vi "运维调试_CODCr.vi"() -> ()   [LabVIEW 2016, in "CODCr库.lvlib"]
uses:
  <vilib>/Utility/miscctls.llb/LVPointTypeDef.ctl
  <vilib>/Plasmionique/MB Master/MB_Master_Serial/MB_Master_Serial.lvclass
  D:/Program Files (x86)/National Instruments/LabVIEW 2016/vi.lib/Plasmionique/MB Master/MB_Master/MB_Master.lvclass
  <vilib>/Plasmionique/MB Master/MB Master.lvlib
  <vilib>/ptbypt/NI_PtbyPt.lvlib
  <vilib>/Utility/config.llb/NI_LVConfig.lvlib
panel:
  in  "加标回收测试":bool
  in  "平行样测试":bool
  in  "定时启动":bool
  out "COM口":string
  in  "空白测试":bool
  in  "隐藏按钮":bool
  in  "写入消解温度时长":bool
  in  "保存KB值":bool
  out "source":string
  in  "标样核查":bool
  out "启动时间":timestamp format="%<%Y/%m/%d %H:%M:%S>T"
  out "主循环次数":i32
  out "status":bool
  out "启动测量模式":T1(ring)
  out "曲线斜率B":sgl format="%#_10g"
  out "曲线斜率K":sgl format="%#_10g"
  out "量程上限":sgl
  out "量程下限":sgl
  out "消解时长":u16
  out "消解温度":u16
  out "测量精度":u16
  out "测量结果":sgl
  out "标样参考值":sgl
  out "量程":u16
  out "工作状态":T1(ring)
  out "仪器时间":timestamp format="%<%X\n%x>T"
  out "关键参数区":T2
  out "状态告警区":T3
  out "测量数据区":T4 {"单位" items=["ug/L", "mg/L", "ppm", "mg/m3", "cm", "ppb", "ug/m3", "%", "nmol/mol", "umol/mol", "MPN/L", "MPN/100ml", "ng/m3", "NTU", "无量纲", "ms/cm", "us/cm", "℃", "mV", "万个/L"]}
  out "系统时间":timestamp format="%<%Y/%m/%d %H:%M:%S>T"
  in  "VISA Resource":refnum<visa-resource-name>="COM9"
  out "Registers":u16[](array[numeric])
  in  "枚举":enum16{"读取", "写入", "读取参数"}(ring)
  in  "停止":bool
  in  "校时":bool
  in  "标样校准":bool
  in  "空白校准":bool
  in  "零点核查":bool
  in  "跨度核查":bool
  in  "水样测试":bool
  in  "返回":bool
  in  "设置":bool
  # "mg/L"
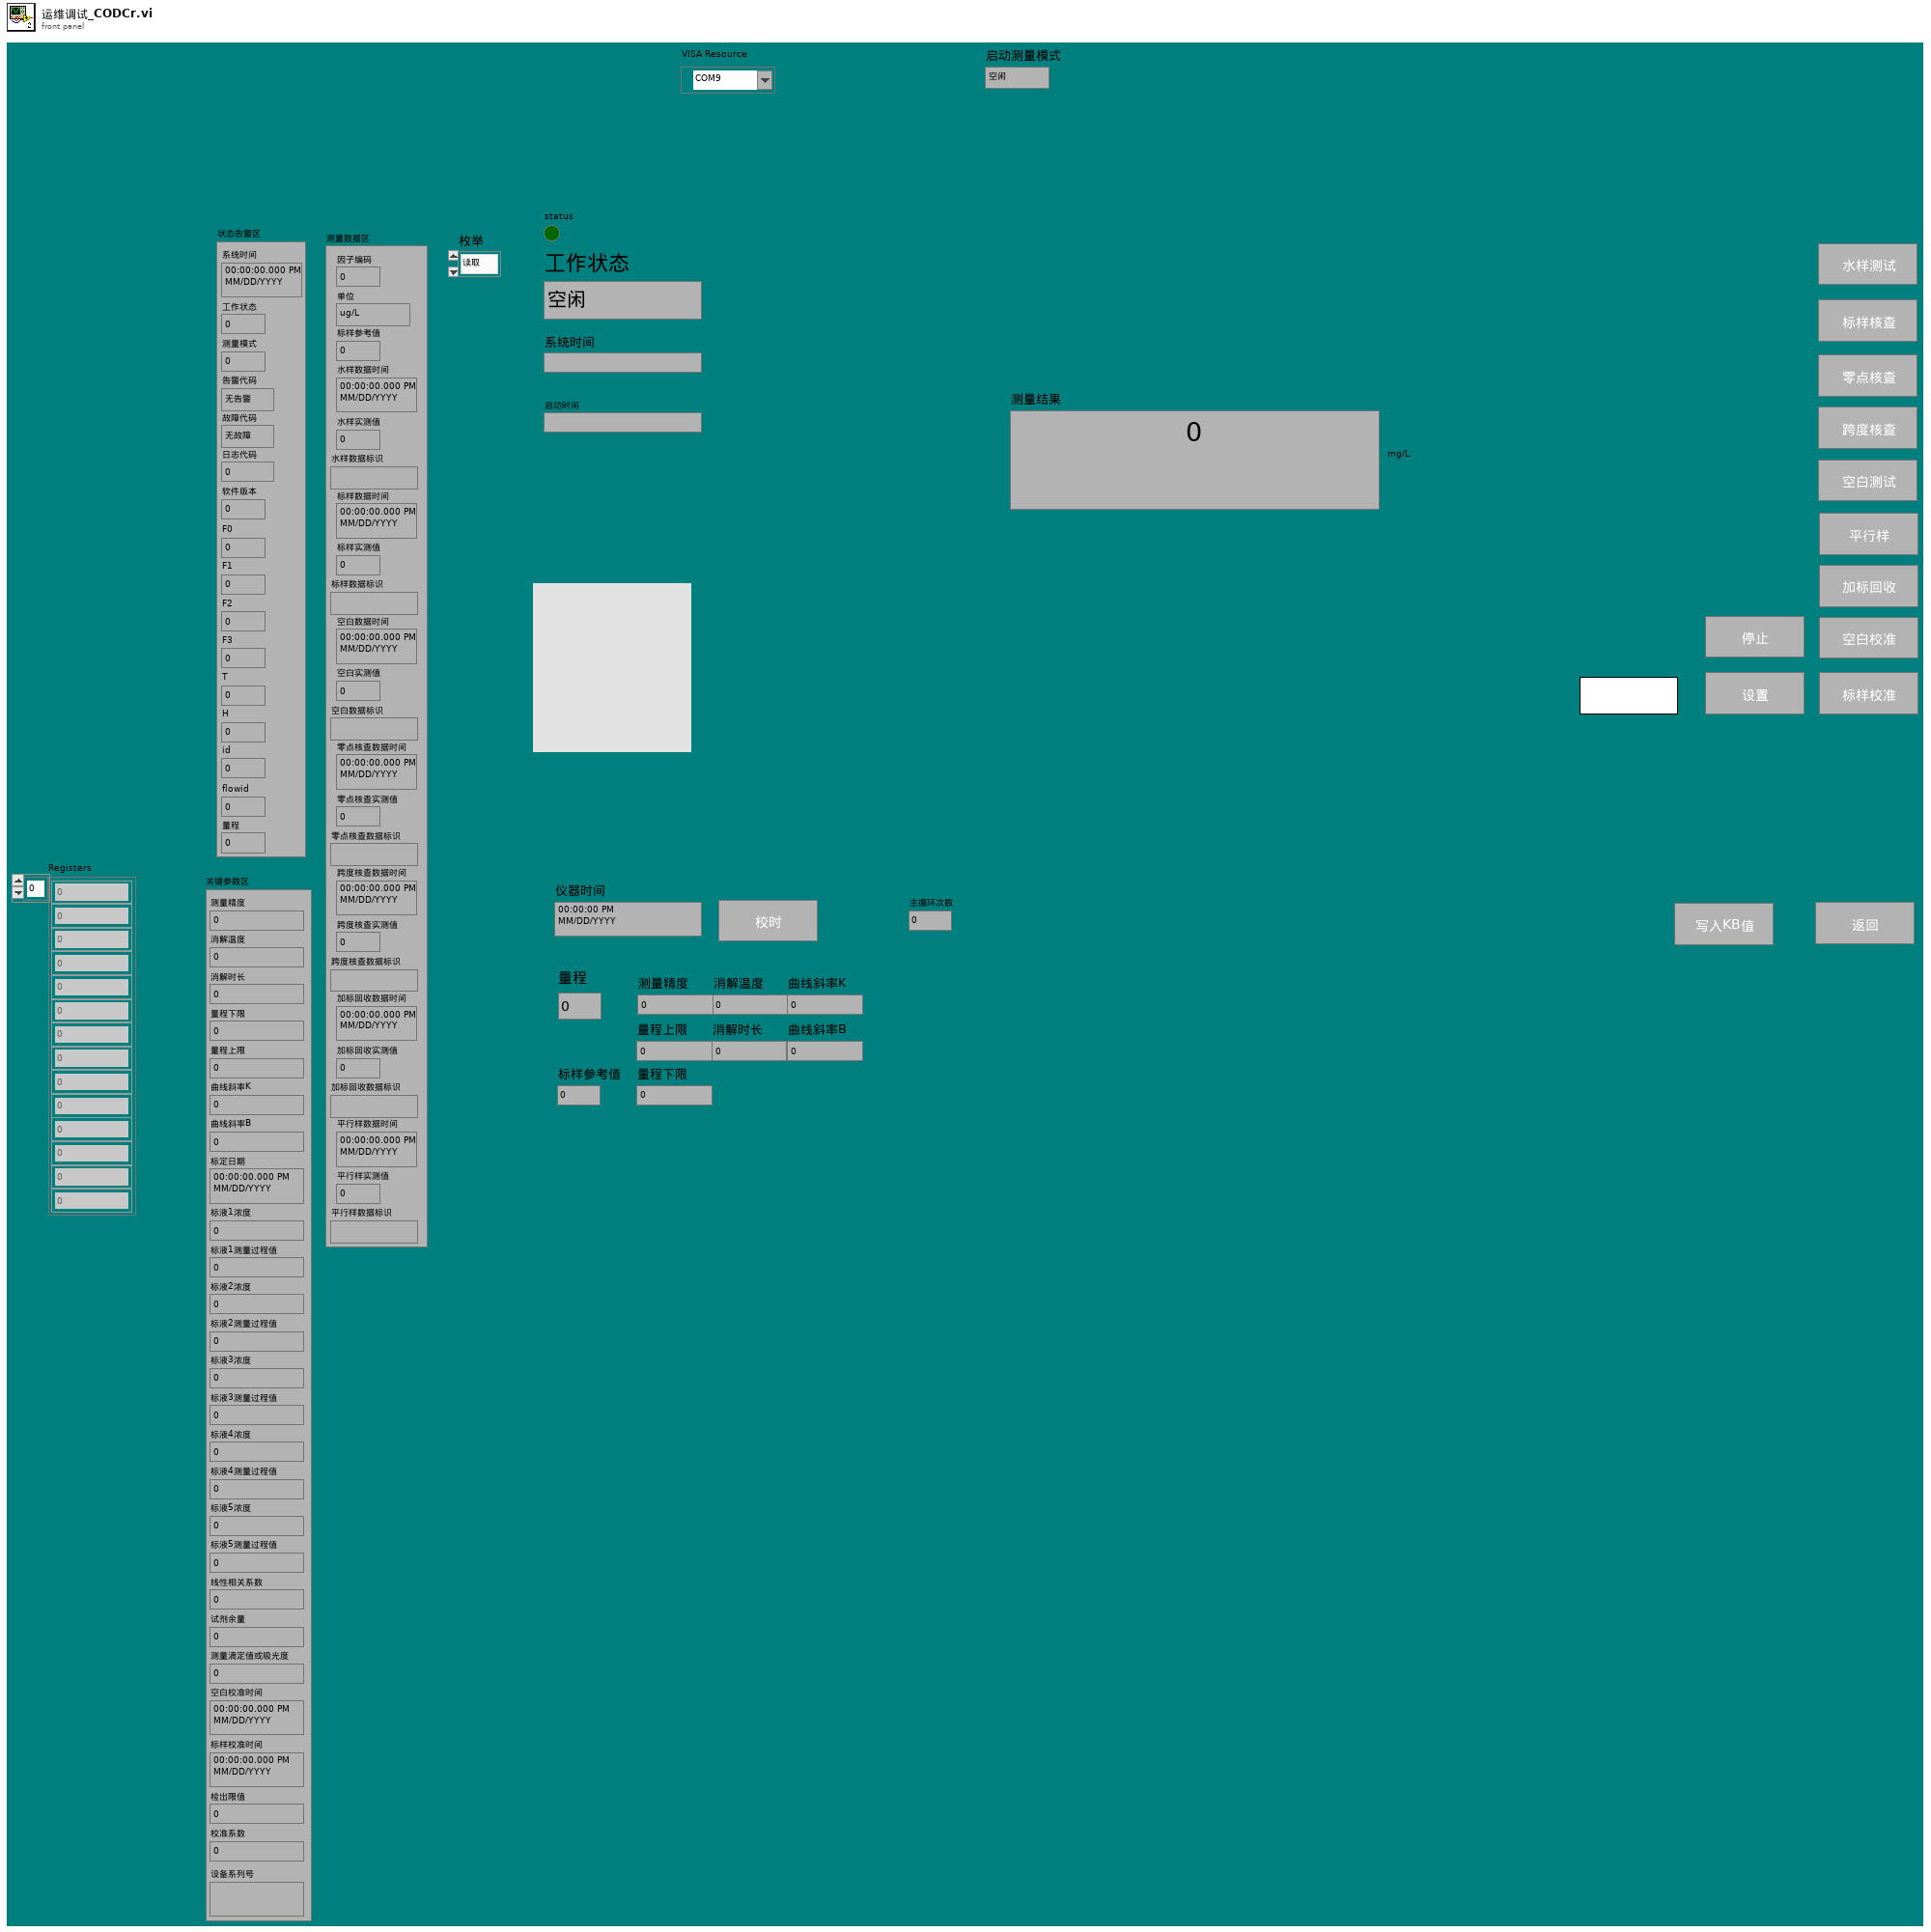
[diagram p1: front panel]
types:
  T1 = enum16{"空闲", "水样测试", "标样核查", "零点核查", "跨度核查", "空白测试", "平行样测试", "加标回收", "空白校准", "标样校准", "初始化（清洗）"}
  T2 = cluster{"测量精度":u16, "消解温度":u16, "消解时长":u16, "量程下限":sgl, "量程上限":sgl, "曲线斜率K":sgl, "曲线斜率B":sgl, "标定日期":timestamp, "标液1浓度":sgl, "标液1测量过程值":sgl, "标液2浓度":sgl, "标液2测量过程值":sgl, "标液3浓度":sgl, "标液3测量过程值":sgl, "标液4浓度":sgl, "标液4测量过程值":sgl, "标液5浓度":sgl, "标液5测量过程值":sgl, "线性相关系数":sgl, "试剂余量":u32, "测量滴定值或吸光度":sgl, "空白校准时间":timestamp, "标样校准时间":timestamp, "检出限值":sgl, "校准系数":sgl, "设备系列号":string}
  T3 = cluster{"系统时间":timestamp, "工作状态":u16, "测量模式":u16, "告警代码":enum16{"无告警", "缺试剂告警", "缺水样告警", "缺蒸馏水告警", "缺标液告警", "仪表漏液告警", "标定异常告警", "超量程告警", "加热异常", "低试剂预警", "超上限告警", "超下限告警", "仪表内部其他异常", "滴定异常告警", "电极异常告警", "量程切换告警", "参数设置告警", "PH电极电位异常", "电导率电极异常", "浊度光度异常", "溶解氧电极异常", "溶解氧光强异常", "温度异常告警", "PH异常告警", "溶解氧异常告警", "电导率异常告警", "浊度异常告警", "叶绿素异常告警", "藻密度异常告警", "蓝绿藻异常告警", "ORP异常告警", "氨氮异常告警", "清洁刷异常告警", "SD卡异常告警", "蓝牙异常告警", "Wifi异常告警", "流程异常告警"}, "故障代码":enum16{"无故障", "电机故障", "温度故障", "通讯故障", "滴定故障"}, "日志代码":u16, "软件版本":u16, "F0":sgl, "F1":sgl, "F2":sgl, "F3":sgl, "T":sgl, "H":sgl, "id":u16, "flowid":u16, "量程":u16}
  T4 = cluster{"因子编码":u32, "单位":u16, "标样参考值":sgl, "水样数据时间":timestamp, "水样实测值":sgl, "水样数据标识":string, "标样数据时间":timestamp, "标样实测值":sgl, "标样数据标识":string, "空白数据时间":timestamp, "空白实测值":sgl, "空白数据标识":string, "零点核查数据时间":timestamp, "零点核查实测值":sgl, "零点核查数据标识":string, "跨度核查数据时间":timestamp, "跨度核查实测值":sgl, "跨度核查数据标识":string, "加标回收数据时间":timestamp, "加标回收实测值":sgl, "加标回收数据标识":string, "平行样数据时间":timestamp, "平行样实测值":sgl, "平行样数据标识":string}
  T5 = cluster{"baud rate (bps)":u32, "stop bits":u16, "parity":u16, "flow control":u16, "timeout":u32, "retries":i32}
  T6 = cluster{"starting address":u16, "number of holding registers":u16}
  T7 = cluster{"测量模式":enum16{"水样测量", "标样核查", "零点核查", "跨度核查", "空白测试", "加标回收", "平行样", "校零", "校标"}}
  T8 = cluster{"仪器测试类型":enum16{"水样测试", "标样核查", "空白测试", "跨度核查"}, "周期设置类型":enum16{"定点启动", "间隔启动"}, "定时功能启用":bool, "定时间隔":dbl, "24H周期设置":bool[]}
  T9 = typedef "LVDateTimeRec.ctl" = cluster{"秒数的小数部分":dbl, "秒":i32, "分":i32, "时":i32, "日":i32, "月":i32, "年":i32, "天数（周）":i32, "天数（年）":i32, "DST":i32}
  T10 = typedef "LVPointTypeDef.ctl" = cluster{"Horizontal":i16, "Vertical":i16}
  T11 = typedef "NI_LVConfig.lvlib/Config Data RefNum.ctl" = refnum<k1>
  T12 = cluster{"运行模式":enum16{"维护模式", "常规模式", "应急模式", "质控模式"}}
  T13 = cluster{"时间标识":timestamp, "监测值":sgl, "单位":u16, "数据标识":string, "因子编码":u32, "标样参考值":sgl, "F0":sgl, "F1":sgl, "F2":sgl, "F3":sgl, "温度":sgl, "湿度":sgl, "量程标识":string}
  T14 = cluster{"系统时间":timestamp, "工作状态":enum16{"空闲", "水样测试", "标样核查", "零点核查", "跨度核查", "空白测试", "平行样测试", "加标回收", "空白校准", "标样校准", "初始化（清洗）"}, "测量模式":enum16{"待机", "连续模式", "周期模式", "定点模式", "受控模式", "手动模式"}, "告警代码":enum16{"无告警", "缺试剂告警", "缺水样告警", "缺蒸馏水告警", "缺标液告警", "仪表漏液告警", "标定异常告警", "超量程告警", "加热异常", "低试剂预警", "超上限告警", "超下限告警", "仪表内部其他异常", "滴定异常告警", "电极异常告警", "量程切换告警", "参数设置告警", "PH电极电位异常", "电导率电极异常", "浊度光度异常", "溶解氧电极异常", "溶解氧光强异常", "温度异常告警", "PH异常告警", "溶解氧异常告警", "电导率异常告警", "浊度异常告警", "叶绿素异常告警", "藻密度异常告警", "蓝绿藻异常告警", "ORP异常告警", "氨氮异常告警", "清洁刷异常告警", "SD卡异常告警", "蓝牙异常告警", "Wifi异常告警", "流程异常告警"}, "故障代码":enum16{"无故障", "电机故障", "温度故障", "通讯故障", "滴定故障"}, "日志代码":u16, "软件版本":u16, "F0":sgl, "F1":sgl, "F2":sgl, "F3":sgl, "T":sgl, "H":sgl, "id":u16, "flowid":u16, "量程":u16}
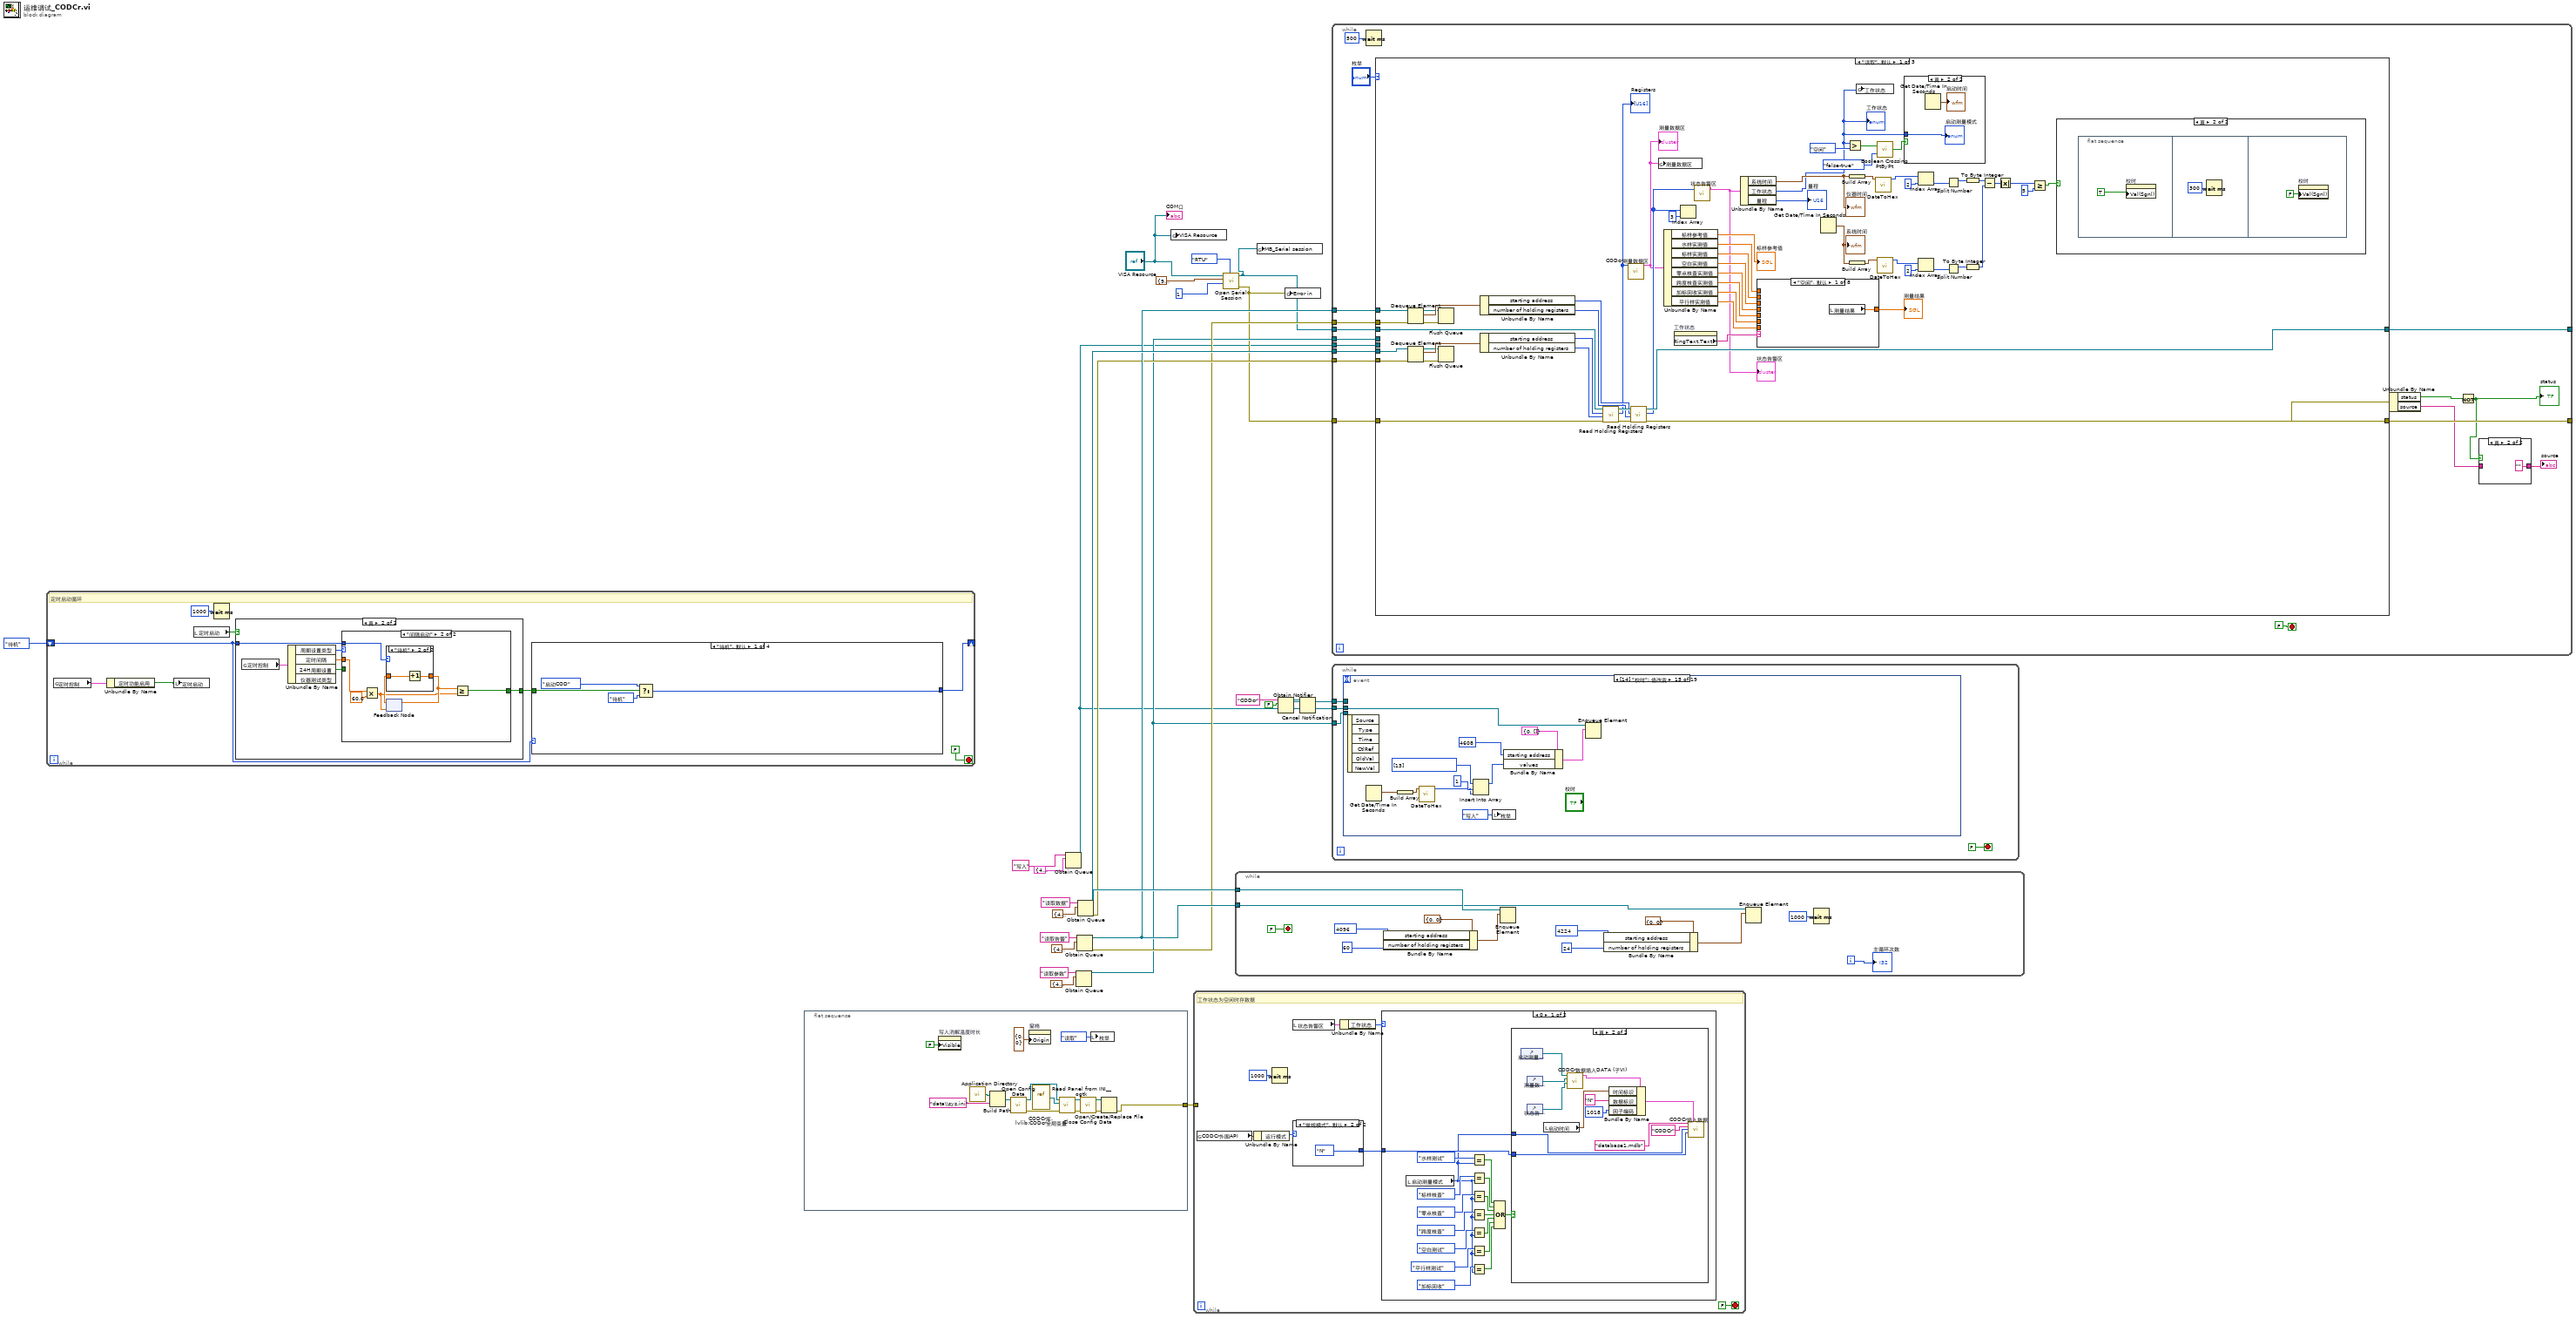
[diagram p0: block diagram]
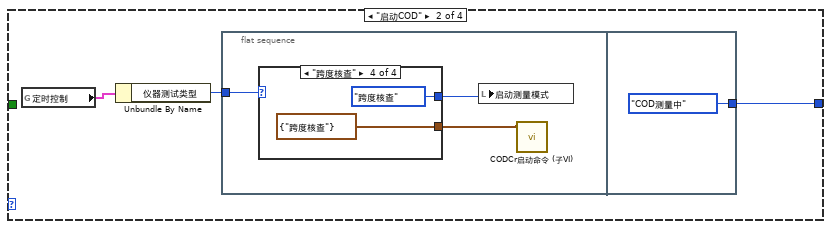
[diagram p2: hidden frame]
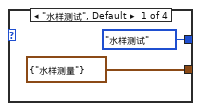
[diagram p3: hidden frame]
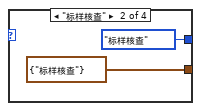
[diagram p4: hidden frame]
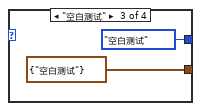
[diagram p5: hidden frame]
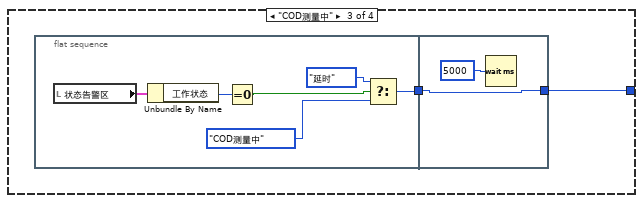
[diagram p6: hidden frame]
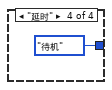
[diagram p7: hidden frame]
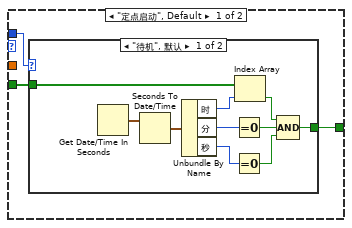
[diagram p9: hidden frame]
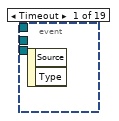
[diagram p12: hidden frame]
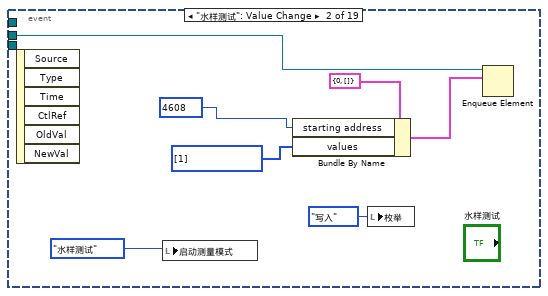
[diagram p13: hidden frame]
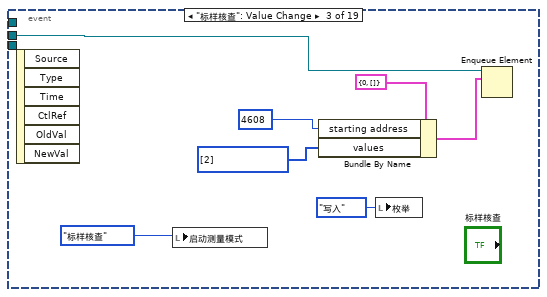
[diagram p14: hidden frame]
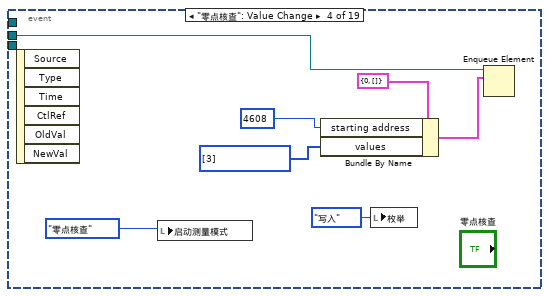
[diagram p15: hidden frame]
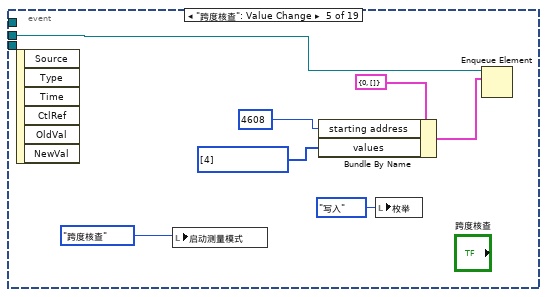
[diagram p16: hidden frame]
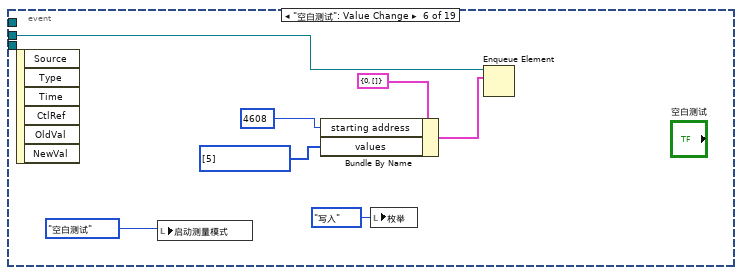
[diagram p17: hidden frame]
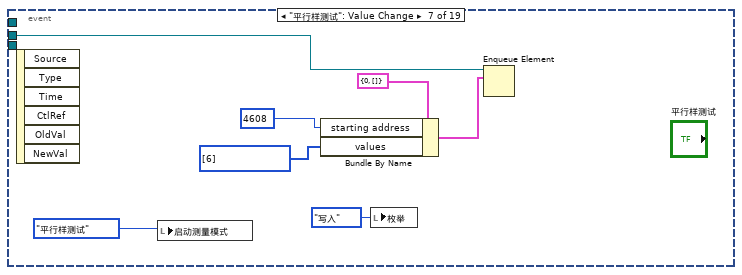
[diagram p18: hidden frame]
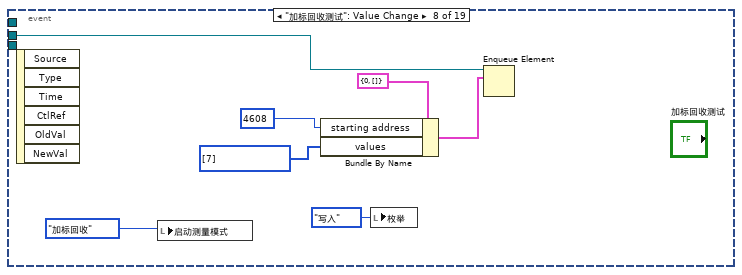
[diagram p19: hidden frame]
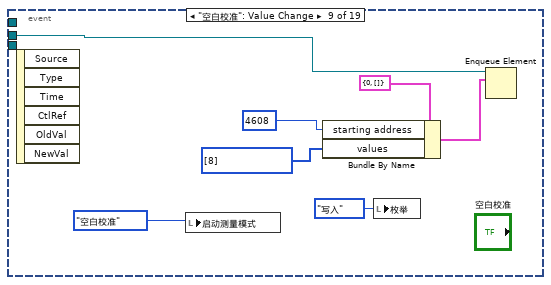
[diagram p20: hidden frame]
diagram:
  n1 = while {
    shift-right: [w32] -> _
    shift-left: enum16{"待机", "启动COD", "COD测量中", "延时"}."待机" -> [w31]
    stop <- FALSE stop-if-true
    # "定时启动循环"
    n2 = global read "CODcr全局变量.vi" "定时控制"() -> (w28:T8)
    n3 = Unbundle By Name(w28) -> ("定时功能启用"=w27:bool)
    n4 = local write "定时启动"(w27) -> ()
    n5 = local read "定时启动"() -> (w29:bool)
    n6 = Wait (ms)(milliseconds to wait=u32 1000 ("等待时间（毫秒）")) -> ()  [unwired: 1 out]
    n7 = case shown="真" w29 {
      tunnel: w31 -> [_ w67]
      tunnel: [_ w66] -> w30
      frame False {
      }
      frame True {
        n8 = global read "CODcr全局变量.vi" "定时控制"() -> (w65:T8)
        n9 = Unbundle By Name(w65) -> ("周期设置类型"=w68:enum16{"定点启动", "间隔启动"}, "定时间隔"=w69:dbl, "24H周期设置"=w70:bool[])  [unwired: 1 out]
        n10 = case shown="\"间隔启动\"" w68 {
          tunnel: w69 -> [_ w87]
          tunnel: w70 -> [w73 _]
          tunnel: w67 -> [w71 w90]
          tunnel: [w72 w85] -> w66
          frame "定点启动", Default {
            n11 = case shown="\"待机\", 默认" w71 {
              tunnel: w73 -> [w81 _]
              tunnel: [w74 _] -> w72
              frame "待机", Default {
                n12 = Get Date/Time In Seconds() -> (seconds since 1Jan1904=w83:timestamp)
                n13 = Seconds To Date/Time(time stamp (now)=w83) -> (date time rec=w82:T9)  [unwired: 1 in]
                n14 = Unbundle By Name(w82) -> ("时"=w80:i32, "分"=w78:i32, "秒"=w79:i32)
                n15 = Equal To 0?(x=w78) -> (x = 0?=w76:bool)
                n16 = Equal To 0?(x=w79) -> (x = 0?=w75:bool)
                n17 = Index Array(array=w81, index=w80) -> (element=w77:bool)
                n18 = Compound Arithmetic op=AND ("复合运算")(w77, w76, w75) -> (w74:bool)
              }
              frame "启动COD" {
              }
            }
          }
          frame "间隔启动" {
            n19 = Multiply(x=w87, y=60.0) -> (x*y=w84:dbl)
            n20 = feedback #1(w84) -> (w89:dbl)
            n21 = case shown="\"待机\"" w90 {
              tunnel: w89 -> [_ w92]
              tunnel: [_ w91] -> w88
              frame Default {
              }
              frame "待机" {
                n22 = Increment(x=w92) -> (x+1=w91:dbl)
              }
            }
            n23 = feedback-in #1(w88) -> ()
            n24 = Greater Or Equal?(x=w88, y=w84) -> (x >= y?=w85:bool)
          }
        }
      }
    }
    n25 = case shown="\"待机\", 默认" w31 {
      tunnel: [w35 w41 w55 enum16{"待机", "启动COD", "COD测量中", "延时"}."待机"] -> w32
      tunnel: w30 -> [w38 _ _ _]
      frame "待机", Default {
        n26 = Select(t=enum16{"待机", "启动COD", "COD测量中", "延时"}."启动COD", s=w38, f=enum16{"待机", "启动COD", "COD测量中", "延时"}."待机") -> (s? t:f=w35:enum16{"待机", "启动COD", "COD测量中", "延时"})
      }
      frame "启动COD" {
        n27 = global read "CODcr全局变量.vi" "定时控制"() -> (w39:T8)
        n28 = Unbundle By Name(w39) -> ("仪器测试类型"=w40:enum16{"水样测试", "标样核查", "空白测试", "跨度核查"})
        n29 = flat-sequence {
          tunnel: w40 -> [w44]
          tunnel: [enum16{"待机", "启动COD", "COD测量中", "延时"}."COD测量中"] -> w41
          frame #0 {
            n30 = case shown="\"跨度核查\"" w44 {
              tunnel: [T7 {"测量模式"=enum."水样测量"} ("启动测量模式") T7 {"测量模式"=enum."标样核查"} ("启动测量模式") T7 {"测量模式"=enum."空白测试"} ("启动测量模式") T7 {"测量模式"=enum."跨度核查"} ("启动测量模式")] -> w43
              tunnel: [T1."水样测试" ("启动测量模式") T1."标样核查" ("启动测量模式") T1."空白测试" ("启动测量模式") T1."跨度核查" ("启动测量模式")] -> w42
              frame "水样测试", Default {
              }
              frame "标样核查" {
              }
              frame "空白测试" {
              }
              frame "跨度核查" {
              }
            }
            n31 = local write "启动测量模式"(w42) -> ()
            n32 = call "CODCr启动命令 (子VI).vi"("启动测量模式"=w43) -> ()  [unwired: 11 in]
          }
          frame #1 {
          }
        }
      }
      frame "COD测量中" {
        n33 = flat-sequence {
          tunnel: [w59] -> w54
          tunnel: [w63] -> w55
          tunnel: w54 -> [w63]
          frame #0 {
            n34 = local read "状态告警区"() -> (w58:T3)
            n35 = Unbundle By Name(w58) -> ("工作状态"=w57:u16)
            n36 = Equal To 0?(x=w57) -> (x = 0?=w56:bool)
            n37 = Select(t=enum16{"待机", "启动COD", "COD测量中", "延时"}."延时", s=w56, f=enum16{"待机", "启动COD", "COD测量中", "延时"}."COD测量中") -> (s? t:f=w59:enum16{"待机", "启动COD", "COD测量中", "延时"})
          }
          frame #1 {
            n38 = Wait (ms)(milliseconds to wait=u32 5000 ("等待时间（毫秒）")) -> ()  [unwired: 1 out]
          }
        }
      }
      frame "延时" {
      }
    }
  }
  n39 = flat-sequence {
    tunnel: [w93] -> w1
    frame #0 {
      n40 = property on="写入消解温度时长" class="Bool"("Visible"=FALSE ("可见")) -> ()  [unwired: 2 in, 2 out]
      n41 = call <vilib>:"Application Directory.vi"() -> ("Application Directory"=w103:path)
      n42 = Build Path(base path=w103, name or relative path="data\\sys.ini" ("名称或相对路径")) -> (appended path=w101:path)
      n43 = call <vilib>:"Open Config Data.vi"("configuration file path"=w101) -> ("error out"=w97:errorcluster, "refnum"=w100:T11)  [unwired: 8 in, 1 out]
      n44 = property on="窗格" class="Pane"("Origin"=T10 {"Horizontal"=0, "Vertical"=0} ("原点")) -> ()  [unwired: 2 in, 2 out]
      n45 = vi-ref "CODCr库.lvlib:CODcr全局变量.vi"() -> (w99:refnum<vi>)
      n46 = call <userlib>:"Read Panel from INI__ogtk.vi"("error in (no error)"=w97, "VI ref"=w99, "refnum"=w100) -> ("error out"=w96:errorcluster, "refnum out"=w98:T11)  [unwired: 7 in]
      n47 = call <vilib>:"Close Config Data.vi"("error in (no error)"=w96, "refnum"=w98) -> ("error out"=w95:errorcluster, "file path"=w94:path)  [unwired: 8 in]
      n48 = local write "枚举"(enum16{"读取", "写入", "读取参数"}."读取" ("枚举")) -> ()
      n49 = Open/Create/Replace File(file path (use dialog)=w94, error in=w95) -> (error out=w93:errorcluster)  [unwired: 4 in, 2 out]
    }
  }
  n50 = Obtain Queue(name (unnamed)="写入" ("名称（未命名）"), element data type=cluster{"starting address":u16, "values":u16[]} {"starting address"=4096, "values"=[]}) -> (queue out=w3:refnum<queue>)  [unwired: 3 in, 2 out]
  n51 = Obtain Queue(name (unnamed)="读取参数" ("名称（未命名）"), element data type=T6 {"starting address"=4096, "number of holding registers"=100}) -> (queue out=w7:refnum<queue>)  [unwired: 3 in, 2 out]
  n52 = Obtain Queue(name (unnamed)="读取告警" ("名称（未命名）"), element data type=T6 {"starting address"=4096, "number of holding registers"=100}) -> (queue out=w16:refnum<queue>, error out=w12:errorcluster)  [unwired: 3 in, 1 out]
  n53 = Obtain Queue(name (unnamed)="读取数据" ("名称（未命名）"), element data type=T6 {"starting address"=4096, "number of holding registers"=100}) -> (queue out=w19:refnum<queue>, error out=w13:errorcluster)  [unwired: 3 in, 1 out]
  n54 = global write "CODcr全局变量.vi" "VISA Resource"("VISA Resource") -> ()
  n55 = while "While循环" {
    tunnel: w1 -> [_]
    stop <- FALSE stop-if-true
    # "工作状态为空闲时存数据"
    n56 = global read "CODCr外部API.vi" "CODCr外围API"() -> (w108:T12)
    n57 = Unbundle By Name(w108) -> ("运行模式"=w107:enum16{"维护模式", "常规模式", "应急模式", "质控模式"})
    n58 = Wait (ms)(milliseconds to wait=u32 1000 ("等待时间（毫秒）")) -> ()  [unwired: 1 out]
    n59 = local read "状态告警区"() -> (w111:T3)
    n60 = case shown="\"常规模式\", 默认" w107 {
      tunnel: [enum16{"N", "M"}."M" ("数据类型") enum16{"N", "M"}."N" ("数据类型")] -> w109
      frame "维护模式" {
      }
      frame "常规模式", Default {
      }
    }
    n61 = Unbundle By Name(w111) -> ("工作状态"=w110:u16)
    n62 = case shown="0" w110 {
      tunnel: w109 -> [w132 _]
      frame 0 {
        n63 = local read "启动测量模式"() -> (w124:T1)
        n64 = Equal?(x=T1."水样测试" ("启动测量模式"), y=w124) -> (x = y?=w123:bool)
        n65 = Equal?(x=T1."标样核查" ("启动测量模式"), y=w124) -> (x = y?=w122:bool)
        n66 = Equal?(x=T1."零点核查" ("启动测量模式"), y=w124) -> (x = y?=w121:bool)
        n67 = Equal?(x=T1."跨度核查" ("启动测量模式"), y=w124) -> (x = y?=w120:bool)
        n68 = Equal?(x=T1."空白测试" ("启动测量模式"), y=w124) -> (x = y?=w119:bool)
        n69 = Equal?(x=T1."平行样测试" ("启动测量模式"), y=w124) -> (x = y?=w118:bool)
        n70 = Equal?(x=T1."加标回收" ("启动测量模式"), y=w124) -> (x = y?=w117:bool)
        n71 = Compound Arithmetic op=OR(w123, w122, w121, w120, w119, w118, w117) -> (w116:bool)
        n72 = case shown="真" w116 {
          tunnel: w124 -> [_ w134]
          tunnel: w132 -> [_ w133]
          frame False {
          }
          frame True {
            n73 = control-ref of="启动测量模式"() -> (w141:refnum<vi>)
            n74 = control-ref of="测量数据区"() -> (w140:refnum<vi>)
            n75 = control-ref of="状态告警区"() -> (w139:refnum<vi>)
            n76 = local read "启动时间"() -> (w144:timestamp)
            n77 = call "CODCr数据插入DATA (子VI).vi"("reference 2"=w139, "reference"=w140, "Enum输入"=w141) -> ("data"=w138:T13)  [unwired: 8 in]
            n78 = Bundle By Name(cluster=w138, "时间标识"=w144, "数据标识"="N", "因子编码"=u32 1018) -> (w137:T13)
            n79 = call "CODCr插入数据.vi"("database"="database1.mdb", "data"=w137, "table"="CODCr", "测量模式"=w134, "数据类型"=w133) -> ()  [unwired: 10 in, 1 out]
          }
        }
      }
      frame 1, Default {
      }
    }
  }
  n80 = call <vilib>:"Open Serial Session.vi"("Mode (RTU)"=enum16{"RTU", "ASCII"}."RTU", "Slave ID"=u8 1, "Serial Config"=T5 {"baud rate (bps)"=9600, "stop bits"=10, "parity"=0, "flow control"=0, "timeout"=1000, "retries"=1}, "VISA Resource"="VISA Resource") -> ("Error out"=w4:errorcluster, "MB_Serial session"=w5:refnum<class "MB_Master_Serial.lvclass">)  [unwired: 6 in]
  n81 = while {
    tunnel: w19 -> [w155]
    tunnel: w16 -> [w146]
    i -> [w145]
    stop <- FALSE stop-if-true
    n82 = Bundle By Name(cluster=T6 {"starting address"=0, "number of holding registers"=0} ("元素"), "starting address"=u16 4096, "number of holding registers"=u16 60) -> (w153:T6)
    n83 = Enqueue Element(queue=w155, element=w153) -> ()  [unwired: 2 in, 3 out]
    n84 = Bundle By Name(cluster=T6 {"starting address"=0, "number of holding registers"=0} ("元素"), "starting address"=u16 4224, "number of holding registers"=u16 24) -> (w147:T6)
    n85 = Enqueue Element(queue=w146, element=w147) -> ()  [unwired: 2 in, 3 out]
    n86 = Wait (ms)(milliseconds to wait=u32 1000 ("等待时间（毫秒）")) -> ()  [unwired: 1 out]
    "主循环次数" <- w145
  }
  n87 = global write "CODcr全局变量.vi" "MB_Serial session"(w5) -> ()
  n88 = Obtain Notifier(name (unnamed)="CODcr" ("名称（未命名）"), notification data type=FALSE) -> (notifier out=w8:refnum<notifier>)  [unwired: 2 in, 2 out]
  n89 = global write "CODcr全局变量.vi" "Error in"(w4) -> ()
  n90 = Cancel Notification(0:w8) -> (8:w9:refnum<notifier>)  [unwired: 1 in, 2 out]
  n91 = while {
    tunnel: w3 -> [w171]
    tunnel: w19 -> [w170]
    tunnel: w16 -> [w169]
    tunnel: w7 -> [w168]
    tunnel: w13 -> [w166]
    tunnel: w12 -> [w165]
    tunnel: w4 -> [w164]
    tunnel: [w162] -> _
    tunnel: w5 -> [w172]
    tunnel: [w167] -> _
    stop <- FALSE stop-if-true
    n92 = Wait (ms)(milliseconds to wait=u32 500 ("等待时间（毫秒）")) -> ()  [unwired: 1 out]
    n93 = case shown="\"读取\", 默认" "枚举" {
      tunnel: w172 -> [w235 w255 w278]
      tunnel: w164 -> [w213 w254 w277]
      tunnel: w171 -> [_ w253 _]
      tunnel: w170 -> [w234 _ _]
      tunnel: w169 -> [w230 _ _]
      tunnel: w168 -> [_ _ w279]
      tunnel: [w212 w249 w267] -> w162
      tunnel: [w198 w250 w268] -> w167
      tunnel: w166 -> [w192 _ _]
      tunnel: w165 -> [w189 _ _]
      frame "读取", Default {
        n94 = Dequeue Element(queue=w230, error in (no error)=w189) -> (queue out=w191:refnum<queue>, element=w229:T6, error out=w190:errorcluster)  [unwired: 1 in, 1 out]
        n95 = Dequeue Element(queue=w234, error in (no error)=w192) -> (queue out=w194:refnum<queue>, element=w233:T6, error out=w193:errorcluster)  [unwired: 1 in, 1 out]
        n96 = Flush Queue(queue=w191, error in (no error)=w190) -> ()  [unwired: 3 out]
        n97 = Flush Queue(queue=w194, error in (no error)=w193) -> ()  [unwired: 3 out]
        n98 = Unbundle By Name(w229) -> ("starting address"=w226:u16, "number of holding registers"=w225:u16)
        n99 = Unbundle By Name(w233) -> ("starting address"=w232:u16, "number of holding registers"=w231:u16)
        n100 = call <vilib>:"Read Holding Registers.vi"("error in (no error)"=w213, "quantity"=w231, "starting address"=w232, "MB session in"=w235) -> ("error out"=w227:errorcluster, "Registers"=w184:u16[], "MB session out"=w228:refnum<class "MB_Master_Serial.lvclass">)  [unwired: 5 in]
        "Registers" <- w184
        n101 = call "CODcr测量数据区.vi"("数组"=w184) -> ("测量数据区"=w178:T4)  [unwired: 10 in]
        "测量数据区" <- w178
        n102 = call <vilib>:"Read Holding Registers.vi"("error in (no error)"=w227, "quantity"=w225, "starting address"=w226, "MB session in"=w228) -> ("error out"=w212:errorcluster, "Registers"=w186:u16[], "MB session out"=w198:refnum<class "MB_Master_Serial.lvclass">)  [unwired: 5 in]
        n103 = global write "CODcr全局变量.vi" "测量数据区"(w178) -> ()
        n104 = Unbundle By Name(w178) -> ("标样参考值"=→"标样参考值":sgl, "水样实测值"=w221:sgl, "标样实测值"=w219:sgl, "空白实测值"=w216:sgl, "零点核查实测值"=w218:sgl, "跨度核查实测值"=w217:sgl, "加标回收实测值"=w214:sgl, "平行样实测值"=w215:sgl)
        n105 = property on="工作状态" class="Enum (严格)"() -> ("RingText.Text"=w222:string)  [unwired: 2 in, 2 out]
        n106 = Index Array(array=w186, index=3 ("索引")) -> ()  [unwired: 1 out]
        n107 = call "状态告警区.vi"("数组"=w186) -> ("状态告警区"=w185:T14)  [unwired: 10 in]
        "状态告警区" <- w185
        n108 = Unbundle By Name(w185) -> ("系统时间"=w199:timestamp, "工作状态"=w179:T1, "量程"=→"量程":u16)
        "仪器时间" <- w199
        "工作状态" <- w179
        n109 = case shown="\"空闲\", 默认" w222 {
          tunnel: w221 -> [_ w240 _ _ _ _ _ _]
          tunnel: [w239 w240 w241 w242 w243 w244 w245 w246] -> w220
          tunnel: w219 -> [_ _ w241 _ _ _ _ _]
          tunnel: w218 -> [_ _ _ w242 _ _ _ _]
          tunnel: w217 -> [_ _ _ _ w243 _ _ _]
          tunnel: w216 -> [_ _ _ _ _ w244 _ _]
          tunnel: w215 -> [_ _ _ _ _ _ w245 _]
          tunnel: w214 -> [_ _ _ _ _ _ _ w246]
          frame "空闲", Default {
            n110 = local read "测量结果"() -> (w239:sgl)
          }
          frame "水样测试" {
          }
          frame "标样核查" {
          }
          frame "零点核查" {
          }
          frame "跨度核查" {
          }
          frame "空白测试" {
          }
          frame "平行样测试" {
          }
          frame "加标回收" {
          }
        }
        "测量结果" <- w220
        n111 = Get Date/Time In Seconds() -> (seconds since 1Jan1904=w200:timestamp)
        "系统时间" <- w200
        n112 = Greater?(x=w179, y=T1."空闲") -> (0:w197:bool)
        n113 = Build Array(w199) -> (w182:timestamp[])
        n114 = Build Array(w200) -> (w183:timestamp[])
        n115 = global write "CODcr全局变量.vi" "工作状态"(w179) -> ()
        n116 = call "DateToHex.vi"("DATE"=w182) -> ("数组"=w181:u16[])  [unwired: 10 in]
        n117 = call <vilib>:"Boolean Crossing PtByPt.vi"("direction"=enum16{"either", "false-true", "true-false"}."false-true", "input"=w197) -> ("crossing"=w196:bool)  [unwired: 1 in]
        n118 = call "DateToHex.vi"("DATE"=w183) -> ("数组"=w180:u16[])  [unwired: 10 in]
        n119 = case shown="真" w196 {
          tunnel: w179 -> [_ w247]
          frame False {
          }
          frame True {
            n120 = Get Date/Time In Seconds() -> (seconds since 1Jan1904=→"启动时间":timestamp)
            "启动测量模式" <- w247
          }
        }
        n121 = Index Array(array=w181, index=2 ("索引")) -> (element=w203:u16)
        n122 = Index Array(array=w180, index=2 ("索引")) -> (element=w202:u16)
        n123 = Split Number(x=w203) -> (hi(x)=w208:u8)  [unwired: 1 out]
        n124 = Split Number(x=w202) -> (hi(x)=w205:u8)  [unwired: 1 out]
        n125 = To Byte Integer(number=w208) -> (8bit integer=w209:i8)
        n126 = To Byte Integer(number=w205) -> (8bit integer=w206:i8)
        n127 = Subtract(x=w209, y=w206) -> (x-y=w207:i8)
        n128 = Absolute Value(x=w207) -> (abs(x)=w210:i8)
        n129 = Greater Or Equal?(x=w210, y=i8 5) -> (x >= y?=w177:bool)
        n130 = case shown="真" w177 {
          frame False {
          }
          frame True {
            n131 = flat-sequence {
              frame #0 {
                n132 = property on="校时" class="Bool (严格)"("Val(Sgnl)"=TRUE ("校时")) -> ()  [unwired: 2 in, 2 out]
              }
              frame #1 {
                n133 = Wait (ms)(milliseconds to wait=u32 300 ("等待时间（毫秒）")) -> ()  [unwired: 1 out]
              }
              frame #2 {
                n134 = property on="校时" class="Bool (严格)"("Val(Sgnl)"=FALSE ("值(信号)")) -> ()  [unwired: 2 in, 2 out]
              }
            }
          }
        }
      }
      frame "写入" {
        n135 = flat-sequence {
          tunnel: w255 -> [w263]
          tunnel: w254 -> [w262]
          tunnel: w253 -> [w259]
          tunnel: [w261] -> w252
          tunnel: [w260] -> w251
          tunnel: w252 -> [w265]
          tunnel: w251 -> [w264]
          tunnel: [w265] -> w250
          tunnel: [w264] -> w249
          frame #0 {
            n136 = Dequeue Element(queue=w259) -> (element=w258:cluster{"starting address":u16, "values":u16[]})  [unwired: 2 in, 3 out]
            n137 = Unbundle By Name(w258) -> ("starting address"=w257:u16, "values"=w256:u16[])
            n138 = call <vilib>:"Write Multiple Registers.vi"("error in (no error)"=w262, "values"=w256, "starting address"=w257, "MB session in"=w263) -> ("error out"=w260:errorcluster, "MB session out"=w261:refnum<class "MB_Master_Serial.lvclass">)  [unwired: 6 in]
          }
          frame #1 {
            n139 = local write "枚举"(enum16{"读取", "写入", "读取参数"}."读取" ("枚举")) -> ()
          }
        }
      }
      frame "读取参数" {
        n140 = local write "枚举"(enum16{"读取", "写入", "读取参数"}."读取" ("枚举")) -> ()
        n141 = Dequeue Element(queue=w279, timeout in ms (-1)=1000 ("超时毫秒(-1)")) -> (element=w286:T6)  [unwired: 1 in, 3 out]
        n142 = Unbundle By Name(w286) -> ("starting address"=w285:u16, "number of holding registers"=w284:u16)
        n143 = call <vilib>:"Read Holding Registers.vi"("error in (no error)"=w277, "quantity"=w284, "starting address"=w285, "MB session in"=w278) -> ("error out"=w281:errorcluster, "Registers"=w283:u16[], "MB session out"=w268:refnum<class "MB_Master_Serial.lvclass">)  [unwired: 5 in]
        n144 = call "关键参数区.vi"("数组"=w283) -> ("关键参数区"=w280:T2)  [unwired: 10 in]
        "关键参数区" <- w280
        n145 = Unbundle By Name(w280) -> ("测量精度"=→"测量精度":u16, "消解温度"=→"消解温度":u16, "消解时长"=→"消解时长":u16, "量程下限"=→"量程下限":sgl, "量程上限"=→"量程上限":sgl, "曲线斜率K"=→"曲线斜率K":sgl, "曲线斜率B"=→"曲线斜率B":sgl)
        n146 = call <vilib>:"Clear Errors.vi"("error in (no error)"=w281) -> ("error out"=w267:errorcluster)  [unwired: 5 in, 1 out]
      }
    }
    n147 = Unbundle By Name(w162) -> ("status"=w163:bool, "source"=w160:string)
    n148 = Not(x=w163) -> (.not. x?=w159:bool)
    "status" <- w159
    n149 = case shown="真" w159 {
      tunnel: w160 -> [w175 _]
      tunnel: [w175 "" ("source")] -> w158
      frame False {
      }
      frame True {
      }
    }
    "source" <- w158
  }
  n150 = while {
    tunnel: w3 -> [w289]
    tunnel: w9 -> [w288]
    tunnel: w7 -> [w287]
    stop <- FALSE stop-if-true
    n151 = event shown="[14] \"校时\": 值改变" {
      selector: _ -> [_ _ _ _ _ _ _ _ _ _ _ _ _ _ _ _ _ _ _]
      dyn-events: _ -> [_ _ _ _ _ _ _ _ _ _ _ _ _ _ _ _ _ _ _]
      timeout: _ -> [_ _ _ _ _ _ _ _ _ _ _ _ _ _ _ _ _ _ _]
      tunnel: w289 -> [_ w297 w300 w307 w314 w321 w328 w335 w342 w349 w357 w375 _ w397 w408 _ _ _ _]
      tunnel: w288 -> [_ _ _ _ _ _ _ _ _ _ w356 _ _ _ _ _ _ _ _]
      tunnel: w287 -> [_ _ _ _ _ _ _ _ _ _ _ _ _ _ _ w412 _ _ _]
      event Timeout {
        n152 = event-data() -> ()  [unwired: 1 in, 2 out]
      }
      event "水样测试": Value Change {
        n153 = event-data() -> ()  [unwired: 1 in, 6 out]
        n154 = local write "启动测量模式"(T1."水样测试" ("启动测量模式")) -> ()
        n155 = Bundle By Name(cluster=cluster{"starting address":u16, "values":u16[]} {"starting address"=0, "values"=[]} ("元素"), "starting address"=u16 4608, "values"=u16[] [1]) -> (w295:cluster{"starting address":u16, "values":u16[]})
        n156 = local write "枚举"(enum16{"读取", "写入", "读取参数"}."写入" ("枚举")) -> ()
        n157 = Enqueue Element(queue=w297, element=w295) -> ()  [unwired: 2 in, 3 out]
      }
      event "标样核查": Value Change {
        n158 = event-data() -> ()  [unwired: 1 in, 6 out]
        n159 = local write "启动测量模式"(T1."标样核查" ("启动测量模式")) -> ()
        n160 = Bundle By Name(cluster=cluster{"starting address":u16, "values":u16[]} {"starting address"=0, "values"=[]} ("元素"), "starting address"=u16 4608, "values"=u16[] [2]) -> (w303:cluster{"starting address":u16, "values":u16[]})
        n161 = local write "枚举"(enum16{"读取", "写入", "读取参数"}."写入" ("枚举")) -> ()
        n162 = Enqueue Element(queue=w300, element=w303) -> ()  [unwired: 2 in, 3 out]
      }
      event "零点核查": Value Change {
        n163 = event-data() -> ()  [unwired: 1 in, 6 out]
        n164 = local write "启动测量模式"(T1."零点核查" ("启动测量模式")) -> ()
        n165 = Bundle By Name(cluster=cluster{"starting address":u16, "values":u16[]} {"starting address"=0, "values"=[]} ("元素"), "starting address"=u16 4608, "values"=u16[] [3]) -> (w310:cluster{"starting address":u16, "values":u16[]})
        n166 = local write "枚举"(enum16{"读取", "写入", "读取参数"}."写入" ("枚举")) -> ()
        n167 = Enqueue Element(queue=w307, element=w310) -> ()  [unwired: 2 in, 3 out]
      }
      event "跨度核查": Value Change {
        n168 = event-data() -> ()  [unwired: 1 in, 6 out]
        n169 = local write "启动测量模式"(T1."跨度核查" ("启动测量模式")) -> ()
        n170 = Bundle By Name(cluster=cluster{"starting address":u16, "values":u16[]} {"starting address"=0, "values"=[]} ("元素"), "starting address"=u16 4608, "values"=u16[] [4]) -> (w317:cluster{"starting address":u16, "values":u16[]})
        n171 = local write "枚举"(enum16{"读取", "写入", "读取参数"}."写入" ("枚举")) -> ()
        n172 = Enqueue Element(queue=w314, element=w317) -> ()  [unwired: 2 in, 3 out]
      }
      event "空白测试": Value Change {
        n173 = event-data() -> ()  [unwired: 1 in, 6 out]
        n174 = local write "启动测量模式"(T1."空白测试" ("启动测量模式")) -> ()
        n175 = Bundle By Name(cluster=cluster{"starting address":u16, "values":u16[]} {"starting address"=0, "values"=[]} ("元素"), "starting address"=u16 4608, "values"=u16[] [5]) -> (w324:cluster{"starting address":u16, "values":u16[]})
        n176 = local write "枚举"(enum16{"读取", "写入", "读取参数"}."写入" ("枚举")) -> ()
        n177 = Enqueue Element(queue=w321, element=w324) -> ()  [unwired: 2 in, 3 out]
      }
      event "平行样测试": Value Change {
        n178 = event-data() -> ()  [unwired: 1 in, 6 out]
        n179 = local write "启动测量模式"(T1."平行样测试" ("启动测量模式")) -> ()
        n180 = Bundle By Name(cluster=cluster{"starting address":u16, "values":u16[]} {"starting address"=0, "values"=[]} ("元素"), "starting address"=u16 4608, "values"=u16[] [6]) -> (w331:cluster{"starting address":u16, "values":u16[]})
        n181 = local write "枚举"(enum16{"读取", "写入", "读取参数"}."写入" ("枚举")) -> ()
        n182 = Enqueue Element(queue=w328, element=w331) -> ()  [unwired: 2 in, 3 out]
      }
      event "加标回收测试": Value Change {
        n183 = event-data() -> ()  [unwired: 1 in, 6 out]
        n184 = local write "启动测量模式"(T1."加标回收" ("启动测量模式")) -> ()
        n185 = Bundle By Name(cluster=cluster{"starting address":u16, "values":u16[]} {"starting address"=0, "values"=[]} ("元素"), "starting address"=u16 4608, "values"=u16[] [7]) -> (w338:cluster{"starting address":u16, "values":u16[]})
        n186 = local write "枚举"(enum16{"读取", "写入", "读取参数"}."写入" ("枚举")) -> ()
        n187 = Enqueue Element(queue=w335, element=w338) -> ()  [unwired: 2 in, 3 out]
      }
      event "空白校准": Value Change {
        n188 = event-data() -> ()  [unwired: 1 in, 6 out]
        n189 = local write "启动测量模式"(T1."空白校准" ("启动测量模式")) -> ()
        n190 = Bundle By Name(cluster=cluster{"starting address":u16, "values":u16[]} {"starting address"=0, "values"=[]} ("元素"), "starting address"=u16 4608, "values"=u16[] [8]) -> (w345:cluster{"starting address":u16, "values":u16[]})
        n191 = local write "枚举"(enum16{"读取", "写入", "读取参数"}."写入" ("枚举")) -> ()
        n192 = Enqueue Element(queue=w342, element=w345) -> ()  [unwired: 2 in, 3 out]
      }
      event "标样校准": Value Change {
        n193 = event-data() -> ()  [unwired: 1 in, 6 out]
        n194 = local write "启动测量模式"(T1."标样校准" ("启动测量模式")) -> ()
        n195 = Bundle By Name(cluster=cluster{"starting address":u16, "values":u16[]} {"starting address"=0, "values"=[]} ("元素"), "starting address"=u16 4608, "values"=u16[] [9]) -> (w352:cluster{"starting address":u16, "values":u16[]})
        n196 = local write "枚举"(enum16{"读取", "写入", "读取参数"}."写入" ("枚举")) -> ()
        n197 = Enqueue Element(queue=w349, element=w352) -> ()  [unwired: 2 in, 3 out]
      }
      event "停止": Value Change {
        n198 = event-data() -> ()  [unwired: 1 in, 6 out]
        n199 = Two Button Dialog(message="确认是否停止！" ("消息")) -> (T button?=w354:bool)  [unwired: 2 in]
        n200 = case shown="真" w354 {
          tunnel: w357 -> [_ w363]
          tunnel: w356 -> [_ w361]
          frame False {
          }
          frame True {
            n201 = Cancel Notification(0:w361) -> (8:w360:refnum<notifier>)  [unwired: 1 in, 2 out]
            n202 = local write "启动测量模式"(T1."空闲" ("启动测量模式")) -> ()
            n203 = Send Notification(notification=TRUE ("通知"), notifier=w360) -> ()  [unwired: 1 in, 2 out]
            n204 = Bundle By Name(cluster=cluster{"starting address":u16, "values":u16[]} {"starting address"=0, "values"=[]} ("元素"), "starting address"=u16 4608, "values"=u16[] [12]) -> (w366:cluster{"starting address":u16, "values":u16[]})
            n205 = local write "枚举"(enum16{"读取", "写入", "读取参数"}."写入" ("枚举")) -> ()
            n206 = Enqueue Element(queue=w363, element=w366) -> ()  [unwired: 2 in, 3 out]
          }
        }
      }
      event "保存KB值": Value Change {
        n207 = event-data() -> ()  [unwired: 1 in, 6 out]
        n208 = local read "曲线斜率B"() -> (w370:sgl)
        n209 = local read "曲线斜率K"() -> (w371:sgl)
        n210 = Build Array(w371, w370) -> (w369:sgl[])
        n211 = call "FloatToHex.vi"("浮点数"=w369) -> ("DCBA整形输出"=w368:u16[])  [unwired: 10 in]
        n212 = Bundle By Name(cluster=cluster{"starting address":u16, "values":u16[]} {"starting address"=0, "values"=[]} ("元素"), "starting address"=u16 4263, "values"=w368) -> (w373:cluster{"starting address":u16, "values":u16[]})
        n213 = Enqueue Element(queue=w375, element=w373) -> ()  [unwired: 2 in, 3 out]
        n214 = local write "枚举"(enum16{"读取", "写入", "读取参数"}."写入" ("枚举")) -> ()
      }
      event "定时启动": Value Change {
        n215 = event-data() -> ()  [unwired: 1 in, 6 out]
        n216 = flat-sequence {
          frame #0 {
            n217 = global read "CODcr全局变量.vi" "定时控制"() -> (w378:T8)
            n218 = call "周期设置.vi"("定时控制参数输入"=w378) -> ("定时控制参数输出"=w377:T8)  [unwired: 10 in]
            n219 = global write "CODcr全局变量.vi" "定时控制"(w377) -> ()
          }
          frame #1 {
            n220 = call <vilib>:"Application Directory.vi"() -> ("Application Directory"=w392:path)
            n221 = Build Path(base path=w392, name or relative path="data\\sys.ini" ("名称或相对路径")) -> (appended path=w390:path)
            n222 = call <vilib>:"Open Config Data.vi"("configuration file path"=w390) -> ("error out"=w386:errorcluster, "refnum"=w389:T11)  [unwired: 8 in, 1 out]
            n223 = vi-ref "CODCr库.lvlib:CODcr全局变量.vi"() -> (w388:refnum<vi>)
            n224 = call <userlib>:"Write Panel to INI__ogtk.vi"("error in (no error)"=w386, "VI ref"=w388, "refnum"=w389) -> ("error out"=w385:errorcluster, "refnum out"=w387:T11)  [unwired: 7 in]
            n225 = call <vilib>:"Close Config Data.vi"("error in (no error)"=w385, "refnum"=w387) -> ("error out"=w380:errorcluster, "file path"=w379:path)  [unwired: 8 in]
            n226 = Open/Create/Replace File(file path (use dialog)=w379, error in=w380) -> (refnum out=w383:refnum<file>, error out=w384:errorcluster)  [unwired: 4 in, 1 out]
            n227 = Flush File(refnum=w383, error in=w384) -> (refnum out=w382:refnum<file>, error out=w381:errorcluster)
            n228 = Close File(refnum=w382, error in=w381) -> ()  [unwired: 2 out]
          }
        }
      }
      event "写入消解温度时长": Value Change {
        n229 = event-data() -> ()  [unwired: 1 in, 6 out]
        n230 = local read "消解时长"() -> (w395:u16)
        n231 = local read "消解温度"() -> (w396:u16)
        n232 = Build Array(w396, w395) -> (w394:u16[])
        n233 = call "WordToHex.vi"("WORD"=w394) -> ("数组"=w393:u16[])  [unwired: 10 in]
        n234 = Bundle By Name(cluster=cluster{"starting address":u16, "values":u16[]} {"starting address"=0, "values"=[]} ("元素"), "starting address"=u16 4257, "values"=w393) -> (w399:cluster{"starting address":u16, "values":u16[]})
        n235 = Enqueue Element(queue=w397, element=w399) -> ()  [unwired: 2 in, 3 out]
      }
      event "校时": Value Change {
        n236 = event-data() -> ()  [unwired: 1 in, 6 out]
        n237 = Get Date/Time In Seconds() -> (seconds since 1Jan1904=w407:timestamp)
        n238 = Build Array(w407) -> (w402:timestamp[])
        n239 = call "DateToHex.vi"("DATE"=w402) -> ("数组"=w401:u16[])  [unwired: 10 in]
        n240 = Insert Into Array(array=u16[] [13] ("values"), index=1 ("索引"), new element=w401) -> (w404:u16[])
        n241 = local write "枚举"(enum16{"读取", "写入", "读取参数"}."写入" ("枚举")) -> ()
        n242 = Bundle By Name(cluster=cluster{"starting address":u16, "values":u16[]} {"starting address"=0, "values"=[]} ("元素"), "starting address"=u16 4608, "values"=w404) -> (w410:cluster{"starting address":u16, "values":u16[]})
        n243 = Enqueue Element(queue=w408, element=w410) -> ()  [unwired: 2 in, 3 out]
      }
      event "设置": Value Change {
        n244 = event-data() -> ()  [unwired: 1 in, 6 out]
        n245 = property on="窗格" class="Pane"("Origin"=T10 {"Horizontal"=0, "Vertical"=728} ("原点")) -> ()  [unwired: 2 in, 2 out]
        n246 = flat-sequence {
          tunnel: w412 -> [w414]
          frame #0 {
            n247 = Bundle By Name(cluster=T6 {"starting address"=0, "number of holding registers"=0} ("元素"), "starting address"=u16 4256, "number of holding registers"=u16 19) -> (w418:T6)
            n248 = Enqueue Element(queue=w414, element=w418) -> ()  [unwired: 2 in, 3 out]
          }
          frame #1 {
            n249 = local write "枚举"(enum16{"读取", "写入", "读取参数"}."读取参数" ("枚举")) -> ()
          }
        }
      }
      event "返回": Value Change {
        n250 = event-data() -> ()  [unwired: 1 in, 6 out]
        n251 = property on="窗格" class="Pane"("Origin"=T10 {"Horizontal"=0, "Vertical"=0} ("原点")) -> ()  [unwired: 2 in, 2 out]
        n252 = property on="写入消解温度时长" class="Bool"("Visible"=FALSE ("可见")) -> ()  [unwired: 2 in, 2 out]
      }
      event "曲线斜率K", "曲线斜率B", "消解温度", "消解时长": Mouse Down {
        n253 = event-data() -> ("CtlRef"=w424:refnum<vi>)  [unwired: 1 in, 7 out]
        n254 = property class="DigNum"(reference=w424) -> (reference out=w425:refnum<vi>, "Value"=w423:variant)  [unwired: 1 in, 1 out]
        n255 = Variant To Data(Variant=w423) -> (data=w422:sgl)  [unwired: 2 in, 1 out]
        n256 = call "CODCR数字键盘.vi"("OldNumber"=w422) -> ("NewNumber"=w426:sgl)
        n257 = property class="DigNum"(reference=w425, "Value"=w426) -> ()  [unwired: 1 in, 2 out]
      }
      event "隐藏按钮": Value Change {
        n258 = event-data() -> ()  [unwired: 1 in, 6 out]
        n259 = property on="写入消解温度时长" class="Bool"("Visible"=TRUE ("可见")) -> ()  [unwired: 2 in, 2 out]
      }
    }
  }
  "COM口" <- "VISA Resource"
